vi "Car_SendUiEvent.vi"(7 "UiEventNames":T1, 8 "ErrorIn":errorcluster, 9 "Data":variant, 11 "Car:Car in":refnum<class "Car.lvclass">) -> (0 "ErrorOut":errorcluster, 3 "Car:Car out":refnum<class "Car.lvclass">)   [LabVIEW 2021, in "Car.lvlib" / "Car.lvclass"]
uses:
  Car.lvclass
  Car_UiCallBackEvents.ctl
  Car.lvclass/Car.ctl
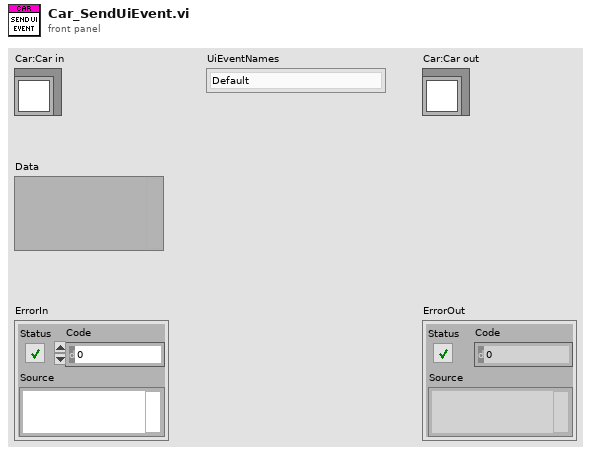
[diagram p1: front panel]
types:
  T1 = typedef "Car.lvlib/Car.lvclass/Car_UiCallBackEvents.ctl" = enum16{"Default", "PersistentDataUpdated"}
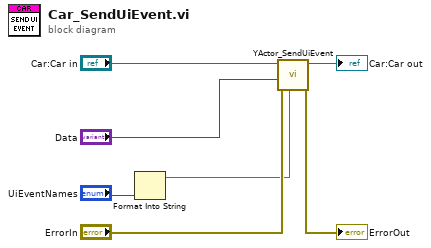
[diagram p0: block diagram]
diagram:
  n1 = Format Into String("UiEventNames") -> (resulting string=w2:string)  [unwired: 3 in, 1 out]
  n2 = call-dynamic "YActor_SendUiEvent.vi"("Event"=w2, "ErrorIn"="ErrorIn", "Data"="Data", "YActorIn"="Car:Car in") -> ("ErrorOut"=→"ErrorOut":errorcluster, "YActorOut"=→"Car:Car out":refnum<class "Car.lvclass">)  [unwired: 6 in]
